vi "Untitled 5.vi"() -> ()   [LabVIEW 2013]
uses:
  <vilib>/Rock Robotics/WPI/Joystick/WPI_JoystickButtonState.ctl
panel:
  out "Buttons":T1
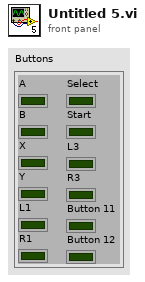
[diagram p1: front panel]
types:
  T1 = typedef "WPI_JoystickButtonState.ctl" = cluster{"A":bool, "B":bool, "X":bool, "Y":bool, "L1":bool, "R1":bool, "Select":bool, "Start":bool, "L3":bool, "R3":bool, "Button 11":bool, "Button 12":bool}
  T2 = typedef "WPI_JoystickDevRef.ctl" = cluster{"Device":T3}
  T3 = typedef "WPI_JoystickDeviceEnum.ctl" = enum16{"USB 1", "USB 2", "USB 3", "USB 4", "Kinect 1", "Kinect 2"}
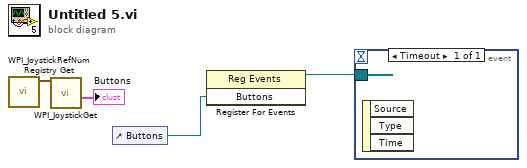
[diagram p0: block diagram]
diagram:
  n1 = call <vilib>:"WPI_JoystickRefNum Registry Get.vi"() -> ("JoystickDevRef"=w4:T2)  [unwired: 10 in, 1 out]
  n2 = call <vilib>:"WPI_JoystickGet.vi"("JoystickDevRef"=w4) -> ("Buttons"=→"Buttons":T1)  [unwired: 4 in, 2 out]
  n3 = control-ref of="Buttons"() -> (w1:refnum<vi>)
  n4 = register-events(w1) -> (reference out=w3:refnum<event-registration>)  [unwired: 2 in, 1 out]
  n5 = event shown="[0] Timeout" {
    selector: w3 -> [_]
    dyn-events: _ -> [_]
    timeout: _ -> [_]
    event Timeout {
      n6 = event-data() -> ()  [unwired: 1 in, 3 out]
    }
  }
